vi "Read stepper.vi"() -> ()   [LabVIEW 2012]
uses:
  <vilib>/Instr/_visa.llb/VISA Configure Serial Port (Instr).vi
panel:
  out "Numeric":i32
  out "read buffer":string
  in  "stop":bool
  out "Waveform Chart":i32(graph)
  in  "Send":bool
  in  "Baud rate":u32=57600
  in  "Serial port":refnum<visa-resource-name>="COM3"
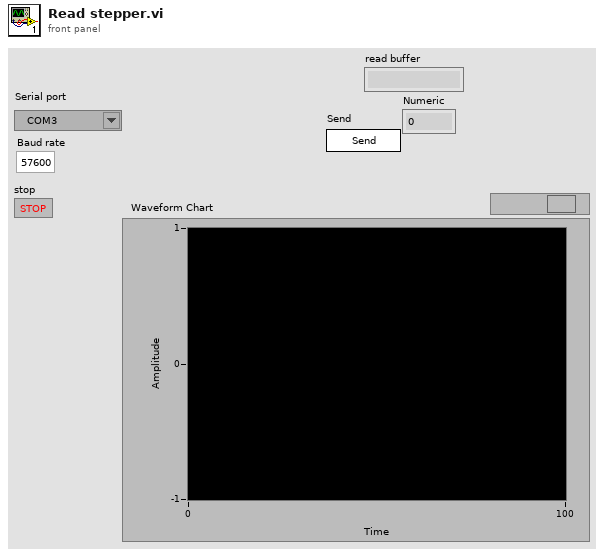
[diagram p1: front panel]
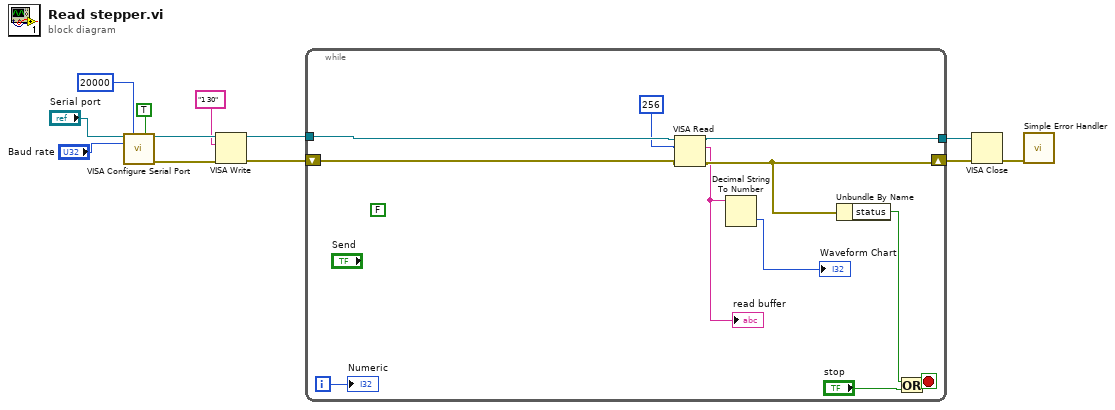
[diagram p0: block diagram]
diagram:
  n1 = call-poly "VISA Configure Serial Port"("VISA resource name"="Serial port", "timeout (10sec)"=u32 20000, "Enable Termination\nChar (T)"=TRUE ("Enable Termination\nChar (T)"), "baud rate (9600)"="Baud rate") -> ("VISA resource name out"=w6:refnum<visa-resource-name>, "error out"=w5:errorcluster)  [unwired: 10 in]
  n2 = VISA Write(VISA resource name=w6, write buffer="1 30", error in (no error)=w5) -> (VISA resource name out=w4:refnum<visa-resource-name>, error out=w3:errorcluster)  [unwired: 1 out]
  n3 = while {
    tunnel: w4 -> [w19]
    shift-right: [w15] -> w9
    shift-left: w3 -> [w16]
    tunnel: [w18] -> w8
    i -> [w13]
    stop <- w22 stop-if-true
    (unwired) FALSE
    n4 = VISA Read(VISA resource name=w19, byte count=u32 256, error in (no error)=w16) -> (VISA resource name out=w18:refnum<visa-resource-name>, read buffer=w14:string, error out=w15:errorcluster)  [unwired: 1 out]
    "read buffer" <- w14
    n5 = Decimal String To Number(string=w14) -> (number=→"Waveform Chart":i32)  [unwired: 2 in, 1 out]
    n6 = Unbundle By Name(w15) -> ("status"=w20:bool)
    n7 = Or(x=w20, y="stop") -> (x .or. y?=w22:bool)
    "Numeric" <- w13
  }
  n8 = VISA Close(VISA resource name=w8, error in (no error)=w9) -> (error out=w7:errorcluster)
  n9 = call <vilib>:"Simple Error Handler.vi"("error in (no error)"=w7) -> ()  [unwired: 4 in, 5 out]
